vi "FP Center and Size.vi"(1 "State":T1(ring)=enum."Standard", 4 "Open?":bool, 5 "OffSets":cluster{"TopOffset":i16, "EdgeOffset":i16}={"TopOffset"=150, "EdgeOffset"=150}, 6 "Mode":T3(ring), 7 "Plane Origin":T2[](array[typedef])=[{"Horizontal"=0, "Vertical"=0}], 8 "error in (no error)":errorcluster, 9 "bottom":i16, 10 "right":i16, 11 "VIRefNum  IN":refnum<vi>) -> (0 "error out":errorcluster, 3 "VIRefNum OUT":refnum<vi>)   [LabVIEW 2019]
uses:
  <vilib>/Utility/miscctls.llb/LVPointTypeDef.ctl
  <vilib>/Utility/miscctls.llb/LVRectTypeDef.ctl
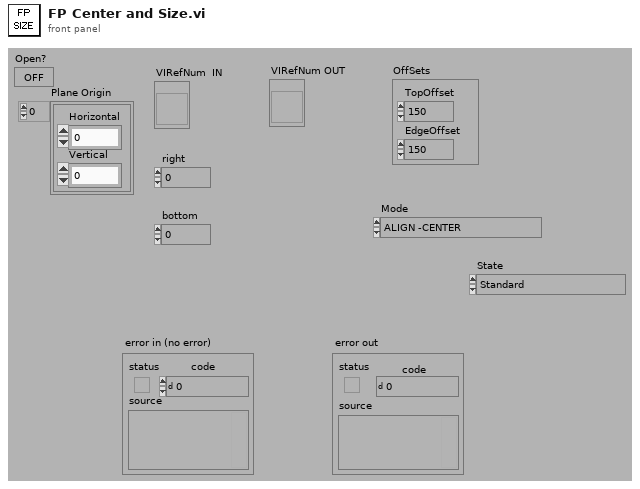
[diagram p1: front panel]
types:
  T1 = enum32{"Invalid", "Standard", "Closed", "Hidden", "Minimized", "Maximized"}
  T2 = typedef "LVPointTypeDef.ctl" = cluster{"Horizontal":i16, "Vertical":i16}
  T3 = enum16{"ALIGN -CENTER", "ALIGN -TOP LEFT", "ALIGN -AS IS", "ALIGN -TOP CENTER", "ALIGN TOP -RIGHT", "ALIGN BOTTOM -Right"}
  T4 = typedef "LVAllMonitorsDisplayTypeDef.ctl" = cluster{"Bounds":cluster{"Left":i16, "Top":i16, "Right":i16, "Bottom":i16}, "Depth":i16}[]
  T5 = typedef "LVRectTypeDef.ctl" = cluster{"Left":i16, "Top":i16, "Right":i16, "Bottom":i16}
  T6 = cluster{"Bounds":cluster{"Left":i16, "Top":i16, "Right":i16, "Bottom":i16}, "Depth":i16}
  T7 = cluster{"left":i16, "top":i16, "right":i16, "bottom":i16}
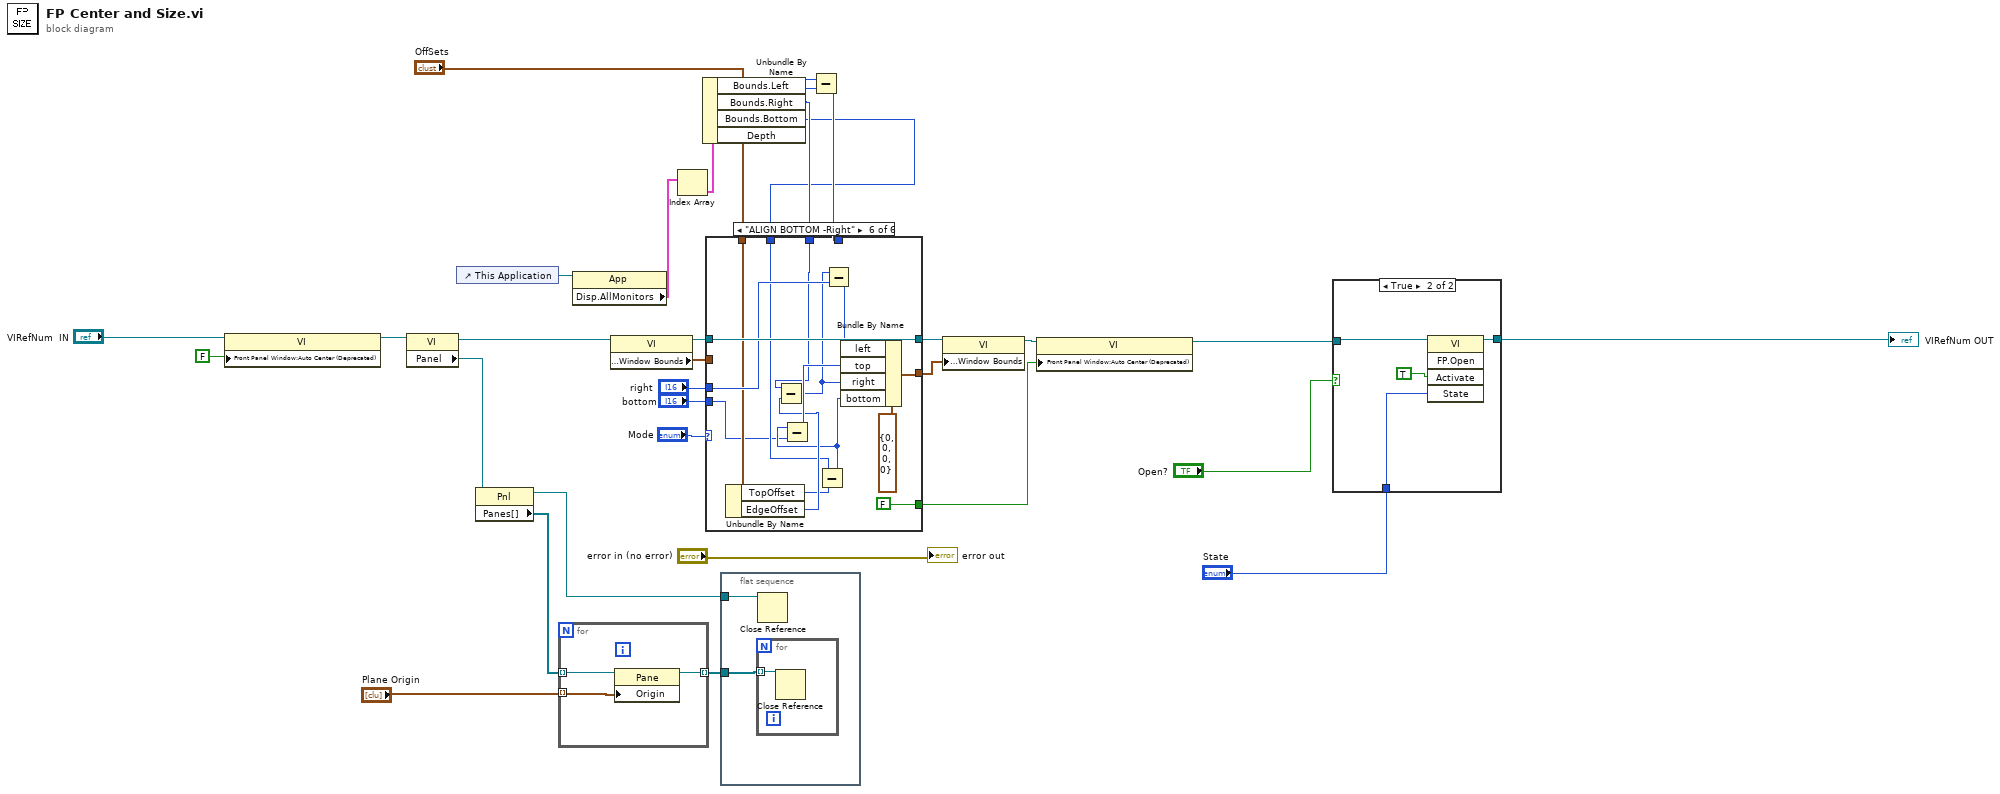
[diagram p0: block diagram]
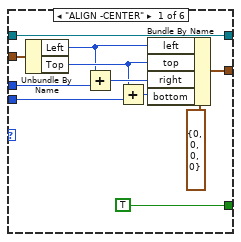
[diagram p3: hidden frame]
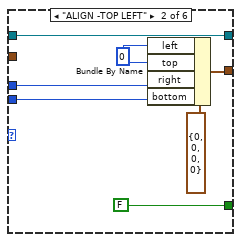
[diagram p4: hidden frame]
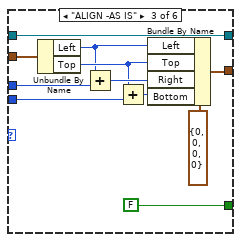
[diagram p5: hidden frame]
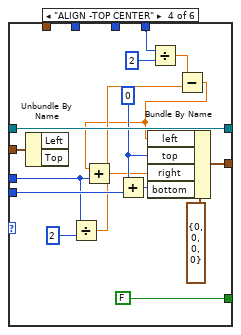
[diagram p6: hidden frame]
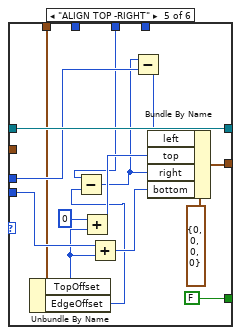
[diagram p7: hidden frame]
diagram:
  n1 = property class="VI"(reference="VIRefNum  IN", "Front Panel Window:Auto Center (Deprecated)"=FALSE ("Front Panel Window:Auto Center")) -> (reference out=w21:refnum<vi>)  [unwired: 1 in, 1 out]
  n2 = property class="VI"(reference=w21) -> (reference out=w20:refnum<vi>, "Panel"=w17:refnum<vi>)  [unwired: 1 in, 1 out]
  n3 = control-ref of="This Application"() -> (w11:refnum<vi>)
  n4 = property class="Pnl"(reference=w17) -> (reference out=w19:refnum<vi>, "Panes[]"=w22:refnum<vi>[])  [unwired: 1 in, 1 out]
  n5 = for {
    tunnel: w22 -> [w34] mode=indexing
    tunnel: [w33] -> w18 mode=indexing
    tunnel: "Plane Origin" -> [w32] mode=indexing
    n6 = property class="Pane"(reference=w34, "Origin"=w32) -> (reference out=w33:refnum<vi>)  [unwired: 1 in, 1 out]
  }
  n7 = property class="App"(reference=w11) -> ("Disp.AllMonitors"=w10:T4)  [unwired: 1 in, 2 out]
  n8 = property class="VI"(reference=w20) -> (reference out=w26:refnum<vi>, "Front Panel Window:Window Bounds"=w28:T5)  [unwired: 1 in, 1 out]
  n9 = Index Array(array=w10) -> (element=w9:T6)  [unwired: 1 in]
  n10 = Unbundle By Name(w9) -> ("Bounds.Left"=w8:i16, "Bounds.Right"=w5:i16, "Bounds.Bottom"=w3:i16)  [unwired: 1 out]
  n11 = flat-sequence {
    tunnel: w19 -> [w36]
    tunnel: w18 -> [w35]
    frame #0 {
      n12 = for {
        tunnel: w35 -> [w37] mode=indexing
        n13 = Close Reference(reference=w37) -> ()  [unwired: 1 in, 1 out]
      }
      n14 = Close Reference(reference=w36) -> ()  [unwired: 1 in, 1 out]
    }
  }
  n15 = Subtract(x=w5, y=w8) -> (x-y=w7:i16)
  n16 = case shown="\"ALIGN BOTTOM -Right\"" "Mode" {
    tunnel: "bottom" -> [w48 w51 w66 w82 w91 w98]
    tunnel: "right" -> [w44 w49 w57 w69 w93 w108]
    tunnel: w28 -> [w41 _ w62 w79 _ _]
    tunnel: [w40 w54 w61 w78 w96 w111] -> w12
    tunnel: w26 -> [w39 w53 w60 w77 w95 w110]
    tunnel: [w39 w53 w60 w77 w95 w110] -> w25
    tunnel: [TRUE FALSE FALSE FALSE FALSE FALSE] -> w24
    tunnel: w7 -> [_ _ _ w72 _ _]
    tunnel: w5 -> [_ _ _ _ w86 w105]
    tunnel: "OffSets" -> [_ _ _ _ w89 w106]
    tunnel: w3 -> [_ _ _ _ _ w102]
    frame "ALIGN -CENTER" {
      n17 = Unbundle By Name(w41) -> ("Left"=w43:i16, "Top"=w45:i16)
      n18 = Add(x=w43, y=w44) -> (x+y=w46:i16)
      n19 = Add(x=w45, y=w48) -> (x+y=w47:i16)
      n20 = Bundle By Name(cluster=T7 {"left"=0, "top"=0, "right"=0, "bottom"=0} ("Front Panel Window:Panel Bounds"), "left"=w43, "top"=w45, "right"=w46, "bottom"=w47) -> (w40:T7)
    }
    frame "ALIGN -TOP LEFT" {
      w50 = i16 0 ("left")
      n21 = Bundle By Name(cluster=T7 {"left"=0, "top"=0, "right"=0, "bottom"=0} ("Front Panel Window:Panel Bounds"), "left"=w50, "top"=w50, "right"=w49, "bottom"=w51) -> (w54:T7)
    }
    frame "ALIGN -AS IS" {
      n22 = Unbundle By Name(w62) -> ("Left"=w56:i16, "Top"=w63:i16)
      n23 = Add(x=w56, y=w57) -> (x+y=w64:i16)
      n24 = Add(x=w63, y=w66) -> (x+y=w65:i16)
      n25 = Bundle By Name(cluster=T5 {"Left"=0, "Top"=0, "Right"=0, "Bottom"=0} ("Front Panel Window:Window Bounds"), "Left"=w56, "Top"=w63, "Right"=w64, "Bottom"=w65) -> (w61:T5)
    }
    frame "ALIGN -TOP CENTER" {
      w75 = i16 0 ("top")
      n26 = Unbundle By Name(w79) -> ()  [unwired: 2 out]
      n27 = Divide(x=w69, y=i16 2) -> (x/y=w70:dbl)
      n28 = Add(x=w75, y=w82) -> (x+y=w81:i16)
      n29 = Divide(x=w72, y=i16 2) -> (x/y=w73:dbl)
      n30 = Subtract(x=w73, y=w70) -> (x-y=w68:dbl)
      n31 = Add(x=w68, y=w69) -> (x+y=w67:dbl)
      n32 = Bundle By Name(cluster=T7 {"left"=0, "top"=0, "right"=0, "bottom"=0} ("Front Panel Window:Panel Bounds"), "left"=w68, "top"=w75, "right"=w67, "bottom"=w81) -> (w78:T7)
    }
    frame "ALIGN TOP -RIGHT" {
      n33 = Unbundle By Name(w89) -> ("TopOffset"=w88:i16, "EdgeOffset"=w85:i16)
      n34 = Subtract(x=w86, y=w85) -> (x-y=w84:i16)
      n35 = Add(x=i16 0 ("left"), y=w88) -> (x+y=w92:i16)
      n36 = Add(x=w91, y=w88) -> (x+y=w90:i16)
      n37 = Subtract(x=w84, y=w93) -> (x-y=w83:i16)
      n38 = Bundle By Name(cluster=T7 {"left"=0, "top"=0, "right"=0, "bottom"=0} ("Front Panel Window:Panel Bounds"), "left"=w83, "top"=w92, "right"=w84, "bottom"=w90) -> (w96:T7)
    }
    frame "ALIGN BOTTOM -Right" {
      n39 = Unbundle By Name(w106) -> ("TopOffset"=w103:i16, "EdgeOffset"=w104:i16)
      n40 = Subtract(x=w105, y=w104) -> (x-y=w101:i16)
      n41 = Subtract(x=w102, y=w103) -> (x-y=w99:i16)
      n42 = Subtract(x=w99, y=w98) -> (x-y=w107:i16)
      n43 = Subtract(x=w101, y=w108) -> (x-y=w100:i16)
      n44 = Bundle By Name(cluster=T7 {"left"=0, "top"=0, "right"=0, "bottom"=0} ("Front Panel Window:Panel Bounds"), "left"=w100, "top"=w107, "right"=w101, "bottom"=w99) -> (w111:T7)
    }
  }
  n45 = property class="VI"(reference=w25, "Front Panel Window:Window Bounds"=w12) -> (reference out=w13:refnum<vi>)  [unwired: 1 in, 1 out]
  n46 = property class="VI"(reference=w13, "Front Panel Window:Auto Center (Deprecated)"=w24) -> (reference out=w6:refnum<vi>)  [unwired: 1 in, 1 out]
  n47 = case shown="True" "Open?" {
    tunnel: w6 -> [w113 w116]
    tunnel: [w113 w115] -> w2
    tunnel: "State" -> [_ w114]
    frame False {
    }
    frame True {
      n48 = invoke class="VI" method="FP.Open"(reference=w116, "Activate"=TRUE ("Activate?"), "State"=w114) -> (reference out=w115:refnum<vi>)  [unwired: 2 in, 4 out]
    }
  }
  "VIRefNum OUT" <- w2
  "error out" <- "error in (no error)"
